vi "LCM of P(x) and Q(x).vi"   [LabVIEW 2020, in "NI_AALPro.lvlib"]
doc: "Computes the least common multiple of two polynomials <B>P(x)</B> and <B>Q(x)</B> with the <B>tolerance</B> you specify. The data types you wire to the <B>P(x)</B> and <B>Q(x)</B> inputs determine the polymorphic instance to use."
uses:
  NI_AALPro.lvlib
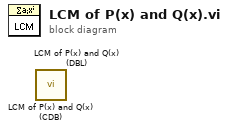
[diagram p0: block diagram]
diagram:
  n1 = call "LCM of P(x) and Q(x) (CDB).vi"() -> ()  [unwired: 10 in, 2 out]
  n2 = call "LCM of P(x) and Q(x) (DBL).vi"() -> ()  [unwired: 10 in, 2 out]
